vi "test Single Write and Read TagDistanceArray to Anchor.vi"(8 "error in (no error)":errorcluster, 11 "TestCase in":refnum<class "AnchorTests.lvclass">) -> (0 "error out":errorcluster, 3 "TestCase out":refnum<class "AnchorTests.lvclass">)   [LabVIEW 2014, in "AnchorTests.lvclass"]
uses:
  AnchorTests.lvclass
  SPLAT/Anchor/Anchor.lvclass
  <vilib>/addons/_JKI Toolkits/VI Tester/TestCase.llb/TestCase.lvclass
  SPLAT/Tag.lvclass
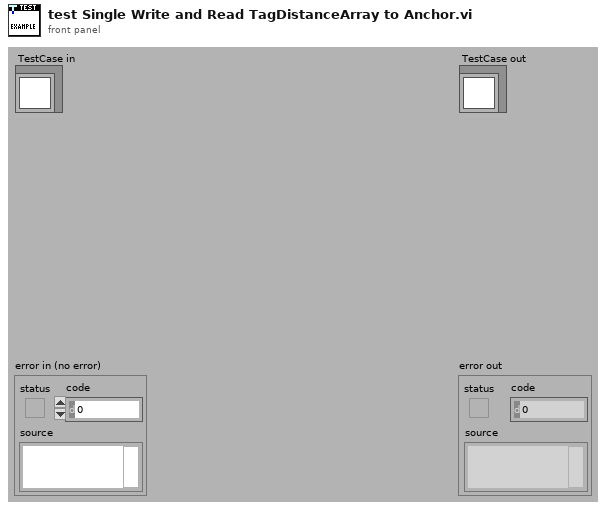
[diagram p1: front panel]
types:
  T1 = cluster{"Tag Out":refnum<class "Tag.lvclass">, "TagY":dbl}
  T2 = cluster{"Tag.lvclass":refnum<class "Tag.lvclass">, "Distance":dbl}[]
  T3 = cluster{"Tag.lvclass":refnum<class "Tag.lvclass">, "Distance":dbl}
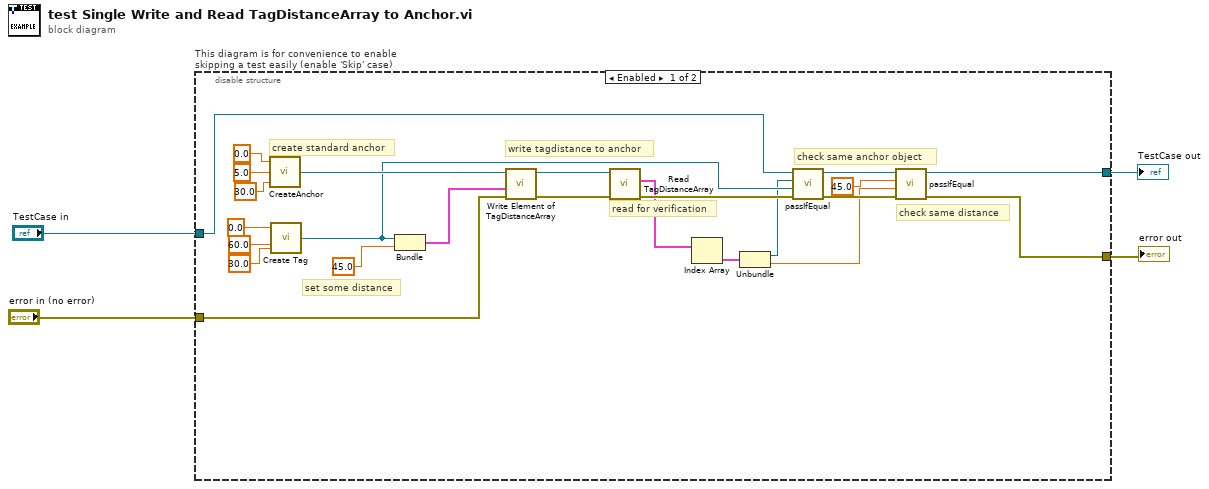
[diagram p0: block diagram]
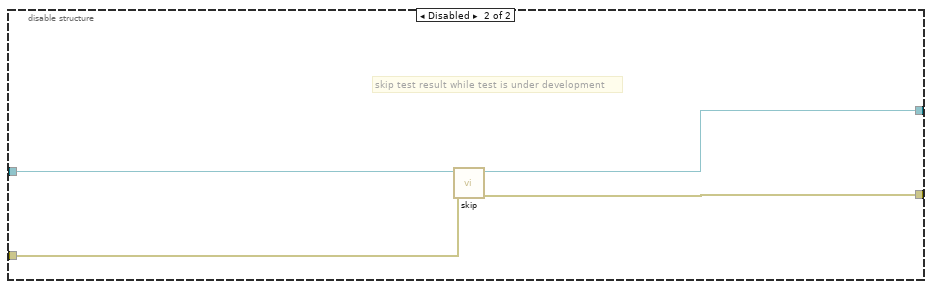
[diagram p2: hidden frame]
diagram:
  n1 = disable-structure "This diagram is for convenience to enable skipping a test easily (enable 'Skip' case)" shown="Enabled" {
    disable-tunnel: "TestCase in" -> [w16 w32]
    disable-tunnel: [w5 w30] -> w1
    disable-tunnel: [w6 w31] -> w3
    disable-tunnel: "error in (no error)" -> [w28 w29]
    frame Enabled {
      # "check same distance"
      # "check same anchor object"
      # "read for verification"
      # "write tagdistance to anchor"
      # "set some distance"
      # "create standard anchor"
      n2 = call "CreateAnchor.vi"("Anchor Y"=30.0, "Anchor X"=5.0, "Anchor ID"=0.0) -> ("Anchor Out"=w21:refnum<class "Anchor.lvclass">)
      n3 = call "Create Tag.vi"("TagY"=30.0, "TagX"=60.0, "TagID"=0.0) -> ("Tag Out"=w13:refnum<class "Tag.lvclass">)
      n4 = Bundle("Tag Out"=w13, "TagY"=45.0) -> (w19:T1)  [unwired: 1 in]
      n5 = call-dynamic "Write Element of TagDistanceArray.vi"("error in (no error)"=w28, "TagDistance"=w19, "Anchor in"=w21) -> ("error out"=w17:errorcluster, "Anchor out"=w18:refnum<class "Anchor.lvclass">)  [unwired: 7 in]
      n6 = call-dynamic "Read TagDistanceArray.vi"("error in (no error)"=w17, "Anchor in"=w18) -> ("error out"=w15:errorcluster, "TagDistanceArray"=w12:T2)  [unwired: 7 in, 1 out]
      n7 = Index Array(array=w12) -> (element=w11:T3)  [unwired: 1 in]
      n8 = Unbundle(w11) -> ("Tag.lvclass"=w10:refnum<class "Tag.lvclass">, "Distance"=w8:dbl)
      n9 = call-dynamic "passIfEqual.vi"("error in (no error)"=w15, "y"=w13, "x"=w10, "TestCase in"=w16) -> ("error out"=w9:errorcluster, "TestCase out"=w14:refnum<class "AnchorTests.lvclass">)  [unwired: 6 in]
      n10 = call-dynamic "passIfEqual.vi"("error in (no error)"=w9, "y"=w8, "x"=45.0 ("Distance"), "TestCase in"=w14) -> ("error out"=w6:errorcluster, "TestCase out"=w5:refnum<class "AnchorTests.lvclass">)  [unwired: 6 in]
    }
    frame Disabled {
      # "skip test result while test is under development"
      n11 = call <vilib>:"skip.vi"("error in (no error)"=w29, "TestCase in"=w32) -> ("error out"=w31:errorcluster, "TestCase out"=w30:refnum<class "AnchorTests.lvclass">)  [unwired: 8 in]
    }
  }
  "error out" <- w3
  "TestCase out" <- w1
